vi "Read_Inputs.vi"(8 "Error In":errorcluster caption="Entrée d'erreur", 9 "Boutons_Appels_Couloir_IHM":bool[](array[boolean]), 10 "Boutons_Destination_Cabine_IHM":bool[](array[boolean]), 11 "Donnees_Globales_IN":T1) -> (0 "Error Out":errorcluster, 1 "Donnees_Globale_Out":T1)   [LabVIEW 2019]
uses:
  Asc_State_Inputs.ctl
  Etat_Asc.ctl
  L298N_Driver/L298N_Ref_Type.ctl
  <vilib>/myRIO/Instrument Drivers/Onboard IO/DIO/typedefs/DIO Reference.ctl
  <vilib>/myRIO/Common/Instrument Driver Framework/Utilities/typedefs/myRIO Generic Hardware Reference.ctl
  <vilib>/myRIO/Common/Instrument Driver Framework/Utilities/typedefs/Hardware Version Enum.ctl
  <vilib>/myRIO/Common/Instrument Driver Framework/Utilities/typedefs/myRIO v1.0 Reference.ctl
  <vilib>/myRIO/Common/Instrument Driver Framework/Utilities/typedefs/Generic FPGA Reference.ctl
  <vilib>/myRIO/Common/Instrument Driver Framework/myRIO v1.0/DIO/typedefs/DIO Channels List.ctl
  <vilib>/myRIO/Common/Instrument Driver Framework/myRIO v1.0/DIO/typedefs/DIO Channels Enum.ctl
  <vilib>/Utility/error.llb/Error Cluster From Error Code.vi
  <vilib>/myRIO/Common/Instrument Driver Framework/myRIO v1.0/DIO/vis/myRIO v1.0 Read DIO.vi
  <vilib>/myRIO/Instrument Drivers/Onboard IO/DIO/DIO.lvlib
panel:
  out "Itération":i32
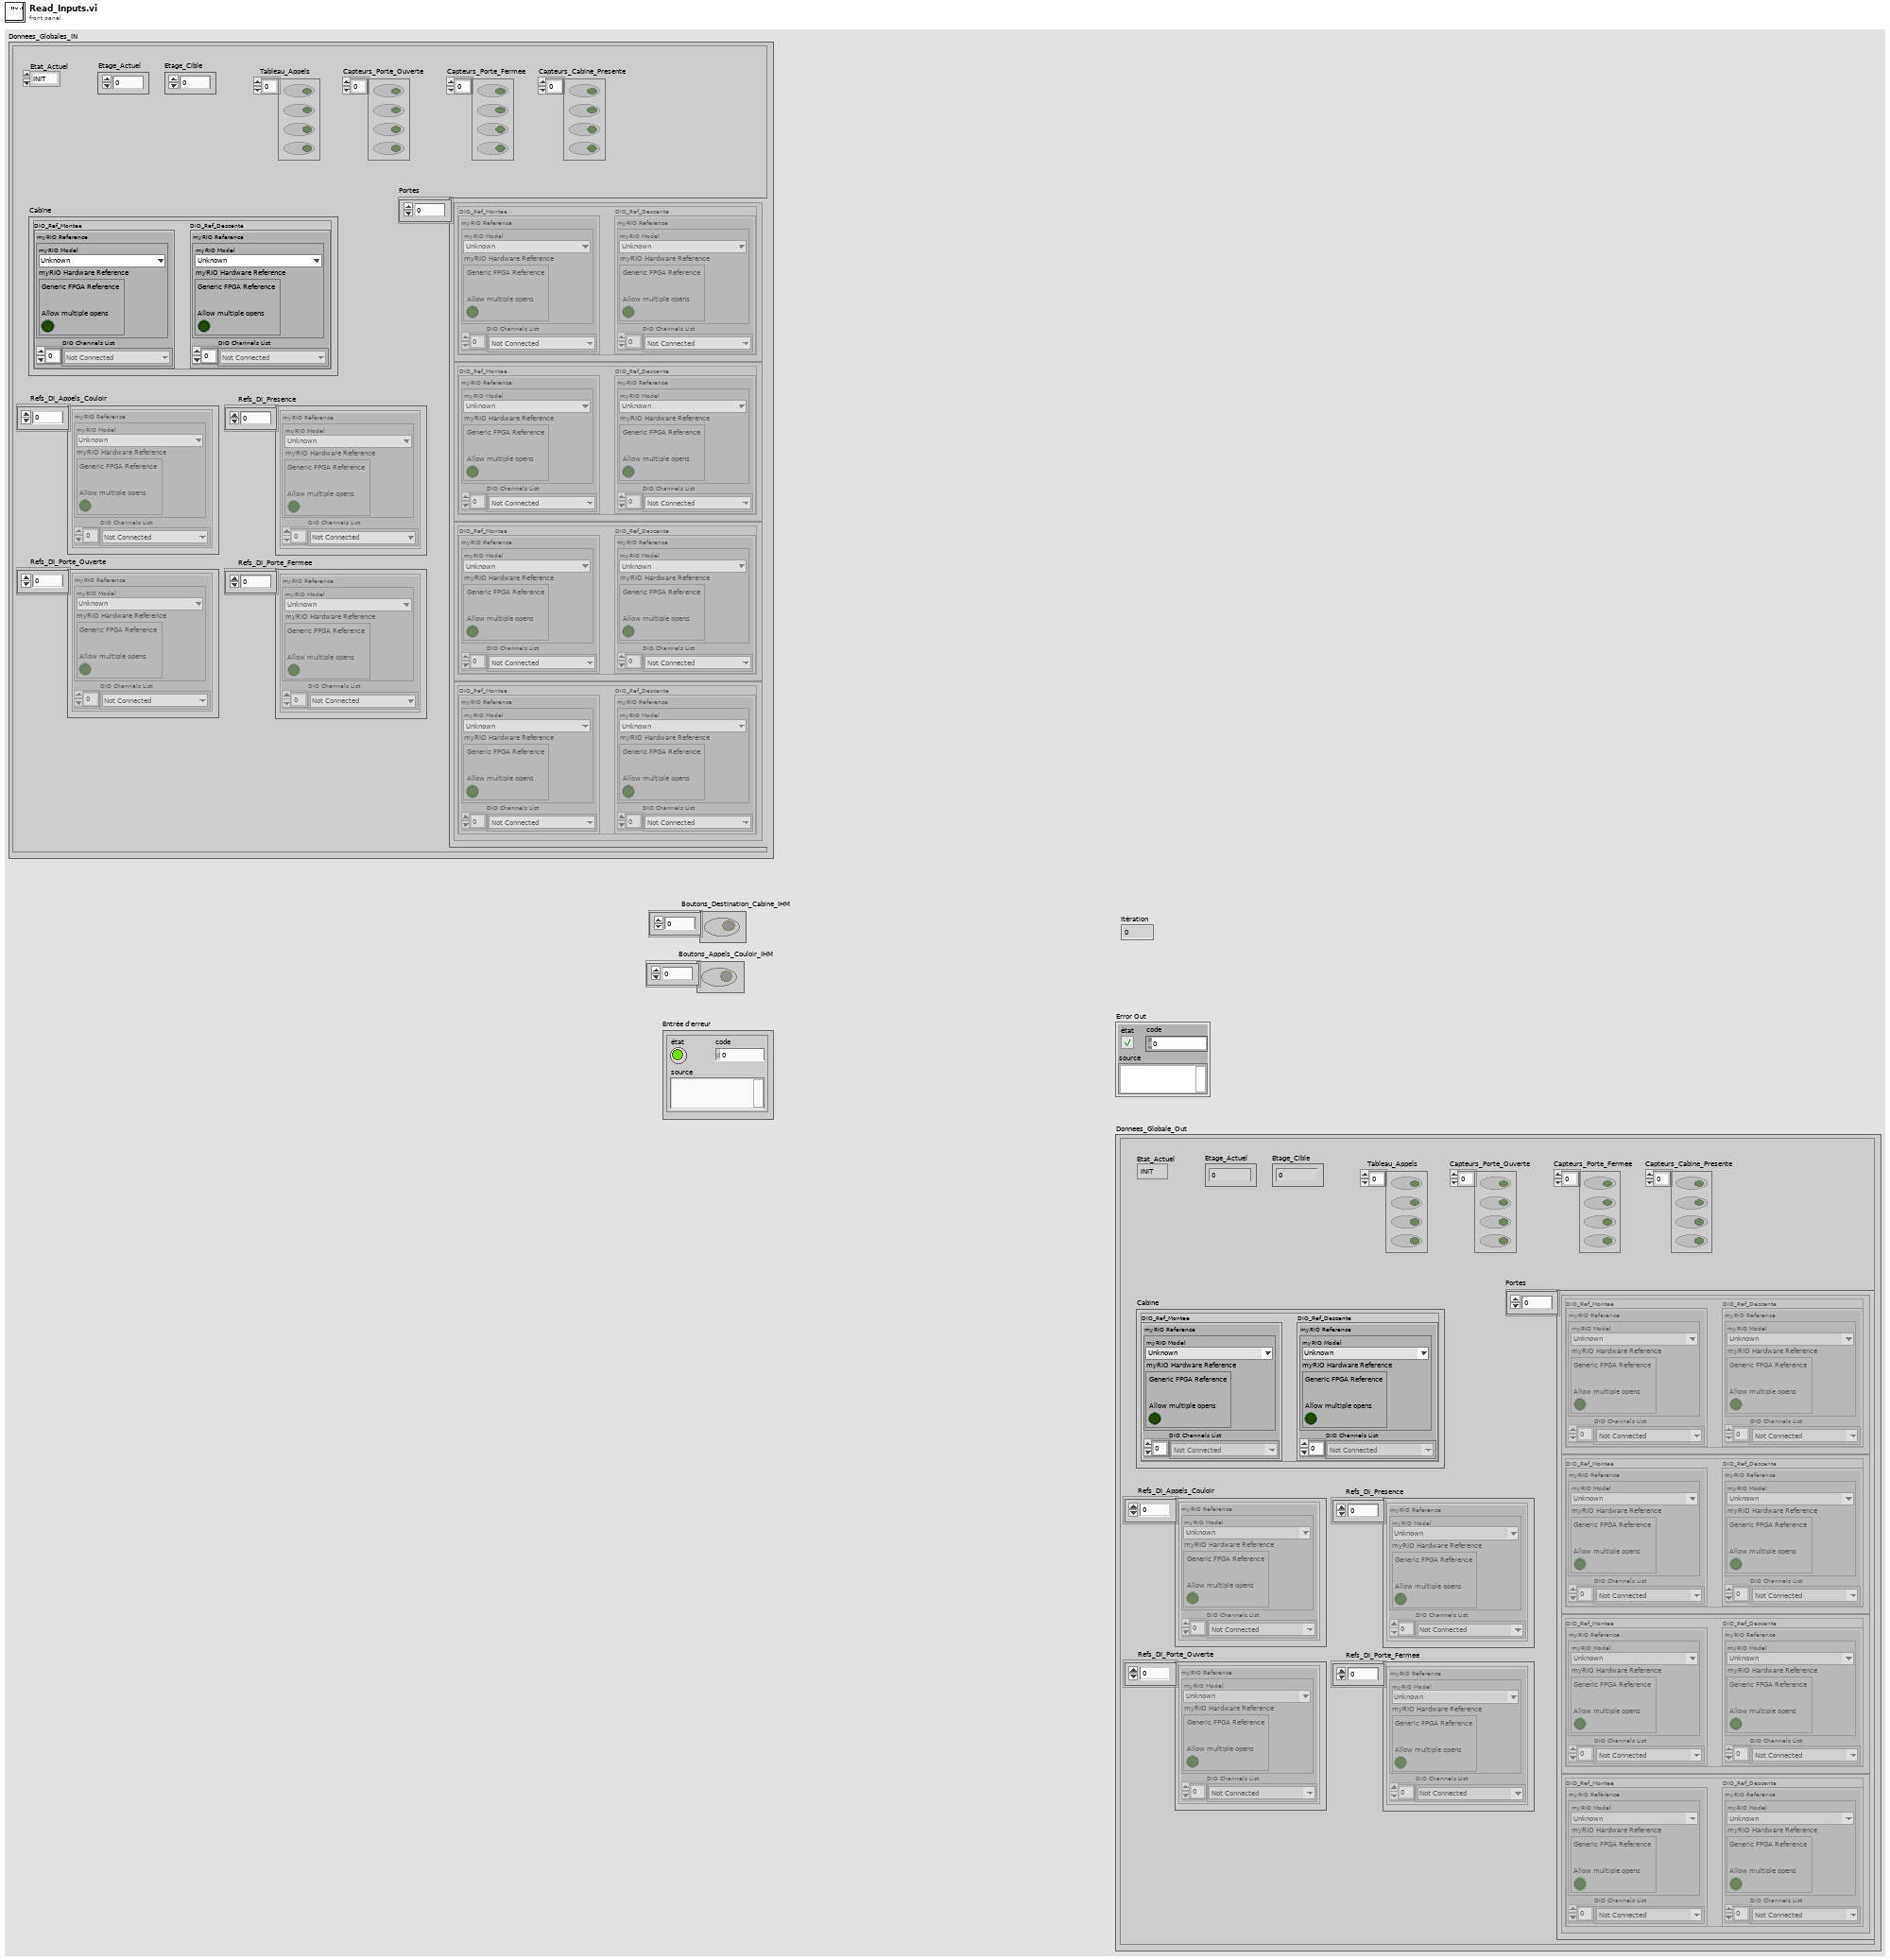
[diagram p1: front panel]
types:
  T1 = typedef "Asc_State_Inputs.ctl" = cluster{"Etage_Actuel":dbl, "Etat_Actuel":T2, "Etage_Cible":dbl, "Tableau_Appels":bool[], "Capteurs_Porte_Ouverte":bool[], "Capteurs_Porte_Fermee":bool[], "Cabine":T3, "Portes":T3[], "Refs_DI_Appels_Couloir":T4[], "Refs_DI_Presence":T4[], "Refs_DI_Porte_Ouverte":T4[], "Refs_DI_Porte_Fermee":T4[], "Capteurs_Cabine_Presente":bool[]}
  T2 = typedef "Etat_Asc.ctl" = enum16{"INIT", "REPOS", "DEPLACEMENT", "OUVERTURE_PORTE", "ATTENTE_TEMPO", "FERMETURE_PORTE", "ARRET_URGENCE"}
  T3 = typedef "L298N_Ref_Type.ctl" = cluster{"DIO_Ref_Montee":T4, "DIO_Ref_Descente":T4}
  T4 = typedef "DIO.lvlib/DIO Reference.ctl" = cluster{"myRIO Reference":T5, "DIO Channels List":T9}
  T5 = typedef "myRIO Generic Hardware Reference.ctl" = cluster{"myRIO Model":T6, "myRIO Hardware Reference":T7}
  T6 = typedef "Hardware Version Enum.ctl" = enum16{"Unknown", "myRIO-1900", "myRIO-1950", "roboRIO", "NI ELVIS RIO CM", "ELVIS III"}
  T7 = typedef "myRIO v1.0 Reference.ctl" = cluster{"Generic FPGA Reference":T8, "Allow multiple opens":bool}
  T8 = typedef "Generic FPGA Reference.ctl" = refnum<k20>
  T9 = typedef "DIO Channels List.ctl" = T10[]
  T10 = typedef "DIO Channels Enum.ctl" = enum16{"Not Connected", "C/DIO0", "C/DIO1", "C/DIO2", "C/DIO3", "C/DIO4", "C/DIO5", "C/DIO6", "C/DIO7", "A/DIO0", "A/DIO1", "A/DIO2", "A/DIO3", "A/DIO4", "A/DIO5", "A/DIO6", "A/DIO7", "A/DIO8", "A/DIO9", "A/DIO10", "A/DIO11", "A/DIO12", "A/DIO13", "A/DIO14", "A/DIO15", "A/DIO16", "A/DIO17", "A/DIO18", "A/DIO19", "B/DIO0", "B/DIO1", "B/DIO2", "B/DIO3", "B/DIO4", "B/DIO5", "B/DIO6", "B/DIO7", "B/DIO8", "B/DIO9", "B/DIO10", "B/DIO11", "B/DIO12", "B/DIO13", "B/DIO14", "B/DIO15", "B/DIO16", "B/DIO17", "B/DIO18", "B/DIO19", "LED0", "LED1", "LED2", "LED3", "Button0", "DIO/DIO0", "DIO/DIO1", "DIO/DIO2", "DIO/DIO3", "DIO/DIO4", "DIO/DIO5", "DIO/DIO6", "DIO/DIO7", "DIO/DIO8", "DIO/DIO9", "SPI/CS0", "SPI/CS1", "SPI/CS2", "SPI/CS3", "LED RADIO (Green)", "LED RADIO (Red)", "LED COMM (Green)", "LED COMM (Red)", "LED MODE (Green)", "LED MODE (Red)"}
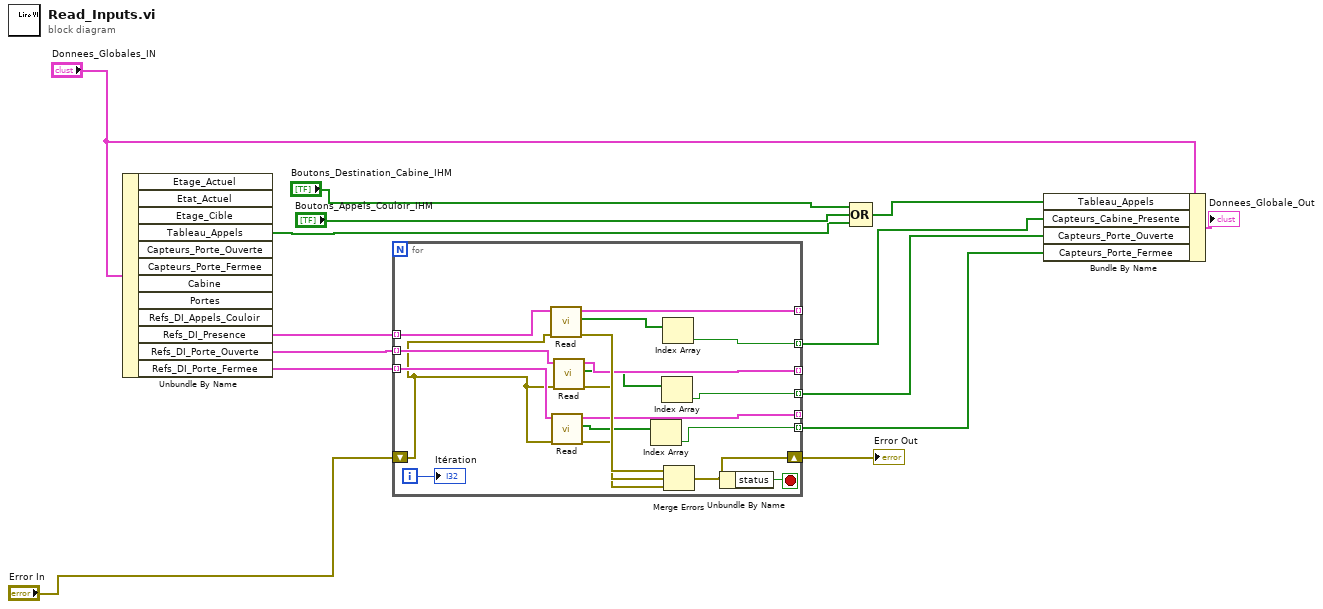
[diagram p0: block diagram]
diagram:
  n1 = Unbundle By Name("Donnees_Globales_IN") -> ("Tableau_Appels"=w7:bool[], "Refs_DI_Presence"=w14:T4[], "Refs_DI_Porte_Ouverte"=w13:T4[], "Refs_DI_Porte_Fermee"=w12:T4[])  [unwired: 8 out]
  n2 = for {
    tunnel: w14 -> [w33] mode=indexing
    tunnel: w13 -> [w32] mode=indexing
    tunnel: w12 -> [w31] mode=indexing
    tunnel: [w27] -> _ mode=indexing
    tunnel: [w26] -> _ mode=indexing
    tunnel: [w25] -> _ mode=indexing
    tunnel: [w23] -> w5 mode=indexing
    tunnel: [w21] -> w4 mode=indexing
    tunnel: [w19] -> w3 mode=indexing
    shift-right: [w16] -> w1
    shift-left: "Error In" -> [w17]
    i -> [w18]
    stop <- w15 stop-if-true
    n3 = call <vilib>:"Read.vi"("error in (no error)"=w17, "DIO Ref In"=w33) -> ("error out"=w30:errorcluster, "Values"=w20:bool[], "DIO Ref Out"=w27:T4)  [unwired: 7 in]
    n4 = call <vilib>:"Read.vi"("error in (no error)"=w17, "DIO Ref In"=w31) -> ("error out"=w28:errorcluster, "Values"=w24:bool[], "DIO Ref Out"=w25:T4)  [unwired: 7 in]
    n5 = call <vilib>:"Read.vi"("error in (no error)"=w17, "DIO Ref In"=w32) -> ("error out"=w29:errorcluster, "Values"=w22:bool[], "DIO Ref Out"=w26:T4)  [unwired: 7 in]
    n6 = Index Array(array=w24) -> (element=w23:bool)  [unwired: 1 in]
    n7 = Index Array(array=w22) -> (element=w21:bool)  [unwired: 1 in]
    n8 = Index Array(array=w20) -> (element=w19:bool)  [unwired: 1 in]
    n9 = Merge Errors(w30, w29, w28) -> (w16:errorcluster)
    n10 = Unbundle By Name(w16) -> ("status"=w15:bool)
    "Itération" <- w18
  }
  "Error Out" <- w1
  n11 = Compound Arithmetic op=OR ("Opérateur arithmétique")("Boutons_Destination_Cabine_IHM", "Boutons_Appels_Couloir_IHM", w7) -> (w9:bool[])
  n12 = Bundle By Name(cluster="Donnees_Globales_IN", "Tableau_Appels"=w9, "Capteurs_Cabine_Presente"=w3, "Capteurs_Porte_Ouverte"=w4, "Capteurs_Porte_Fermee"=w5) -> (→"Donnees_Globale_Out":T1)
